vi "ImageGetScanMoveType.vi"(8 "error in (no error)":errorcluster, 11 "Image in":refnum<class "Image.lvclass">) -> (0 "error out":errorcluster, 3 "Image out":refnum<class "Image.lvclass">)   [LabVIEW 2012, in "Image.lvclass"]
uses:
  classes/Image.lvclass
  classes/Image.lvclass/Image.ctl
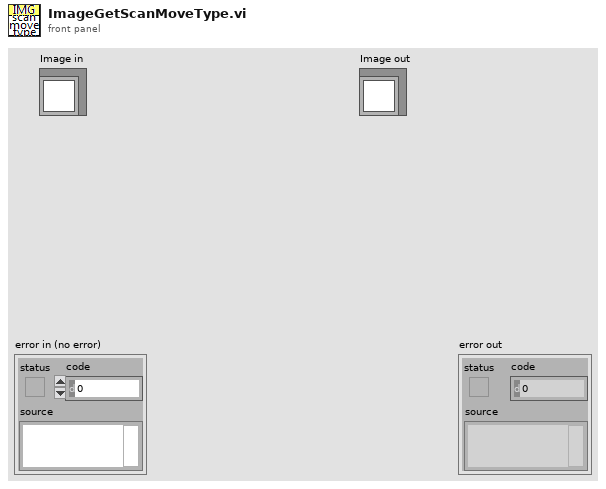
[diagram p1: front panel]
types:
  T1 = typedef "ScanMode.ctl" = enum16{"None", "Continuous", "Point Scan (CH3 cursor)", "Point Scan Move (CH3 cursor)", "Grab", "Grab Move Stage", "Grab Move Z-stage", "Cont. Move Z-stage", "Spec Move Stage", "Spec Move Cont", "Surf Calib"}
  T2 = typedef "DetectorType.ctl" = enum16{"PMT", "SpectraWiz"}
  T3 = typedef "Move Type.ctl" = enum16{"None", "Continuous", "Discrete"}
  T4 = typedef "Scan Type.ctl" = enum16{"None", "Point", "Full Image Continuous", "Full Image Grab"}
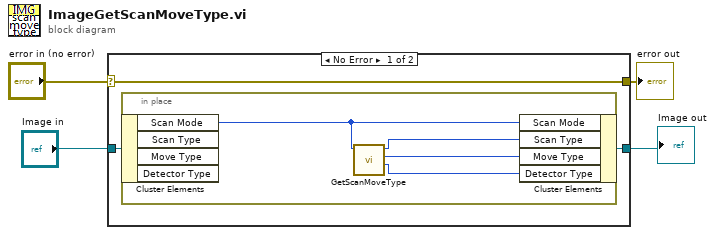
[diagram p0: block diagram]
diagram:
  n1 = case shown="No Error" "error in (no error)" {
    selector: "error in (no error)" -> [w7 w13]
    tunnel: [w7 w13] -> w3
    tunnel: [w5 w12] -> w1
    tunnel: "Image in" -> [w6 w12]
    frame No Error {
      n2 = in-place {
        n3 = in-place-cluster #1(w6) -> ("Scan Mode"=w11:T1)  [unwired: 3 out]
        n4 = call "GetScanMoveType.vi"("Scan Mode"=w11) -> ("Detector"=w8:T2, "Move Type"=w9:T3, "Scan Type"=w10:T4)  [unwired: 8 in]
        n5 = in-place-cluster #1("Scan Mode"=w11, "Scan Type"=w10, "Move Type"=w9, "Detector Type"=w8) -> (w5:refnum<class "Image.lvclass">)
      }
    }
    frame Error {
    }
  }
  "error out" <- w3
  "Image out" <- w1
